vi "QTrkGetProfilingReport.vi"(11 "QTrk Instance":T1) -> (2 "report":string, 3 "QTrk Instance (out)":T1)   [LabVIEW 2011]
uses:
  QTrkInstance.ctl
  QTrkDLL.vi
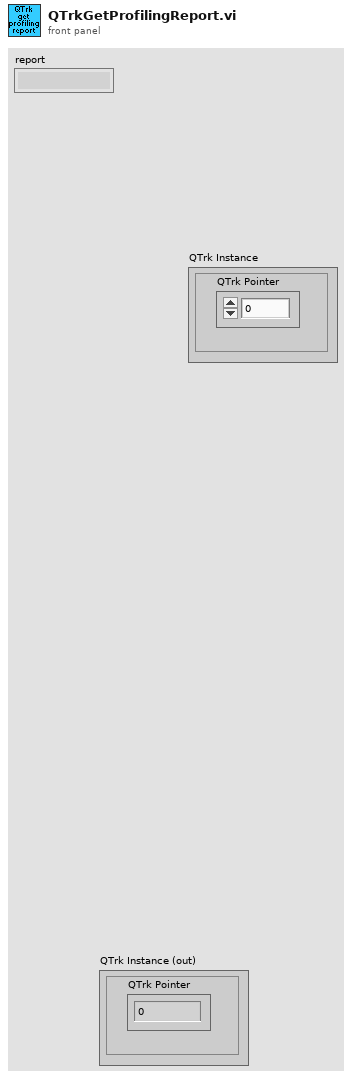
[diagram p1: front panel]
types:
  T1 = typedef "QTrkInstance.ctl" = cluster{"QTrk Pointer":u64}
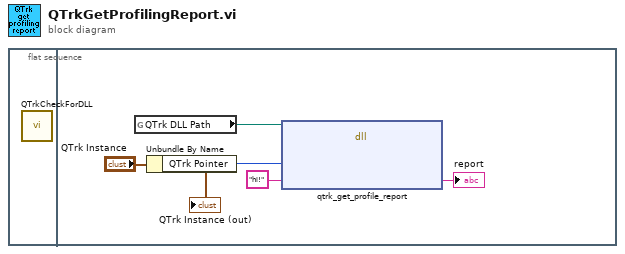
[diagram p0: block diagram]
diagram:
  n1 = flat-sequence {
    frame #0 {
      n2 = call "QTrkCheckForDLL.vi"() -> ()  [unwired: 12 in]
    }
    frame #1 {
      n3 = global read "QTrkDLL.vi" "QTrk DLL Path"() -> (w3:path)
      n4 = Unbundle By Name("QTrk Instance") -> ("QTrk Pointer"=w1:u64)
      n5 = dll-call lib="D:/jcnossen1/cudaqi-tracker/bin/jtrkd-labview.dll" fn="qtrk_get_profile_report"(path in=w3, "qtrk"=w1, "report"="hi!") -> ("report"=→"report":string)  [unwired: 4 in, 2 out]
      "QTrk Instance (out)" <- "QTrk Instance"
    }
  }
